vi "MakeError.vi"(8 "error in":errorcluster, 9 "String":string, 10 "Boolean":bool, 11 "Numeric":dbl) -> (0 "error out":errorcluster)   [LabVIEW 2020]
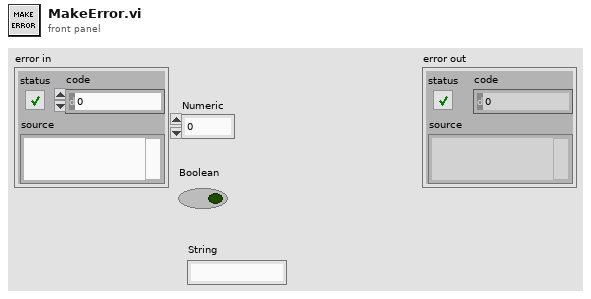
[diagram p1: front panel]
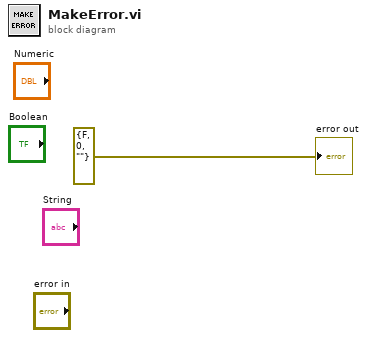
[diagram p0: block diagram]
diagram:
  "error out" <- errorcluster {"status"=FALSE, "code"=0, "source"=""} ("error constant")
